vi "弹窗-创建设备选项.vi"() -> (3 "初始化的属性":T1[](array[typedef]))   [LabVIEW 2017]
panel:
  in  "发现的网络探头":string[](array[string])
  in  "标志-确定创建?":bool
  in  "发现的串口探头":u8[](array[numeric])
  in  "超时":i32
  out "扫描结果":string caption="新的设备"
  out "扫描进度":string
  in  "批量创建":u8=1 min=1 max=10
  in  "扫描探头":bool
  in  "探头类型":enum16{"网络探头", "串口探头"}(ring)
  in  "确定":bool
  in  "取消":bool
  out "信号-关闭窗口":bool=TRUE
  # "创建选项"
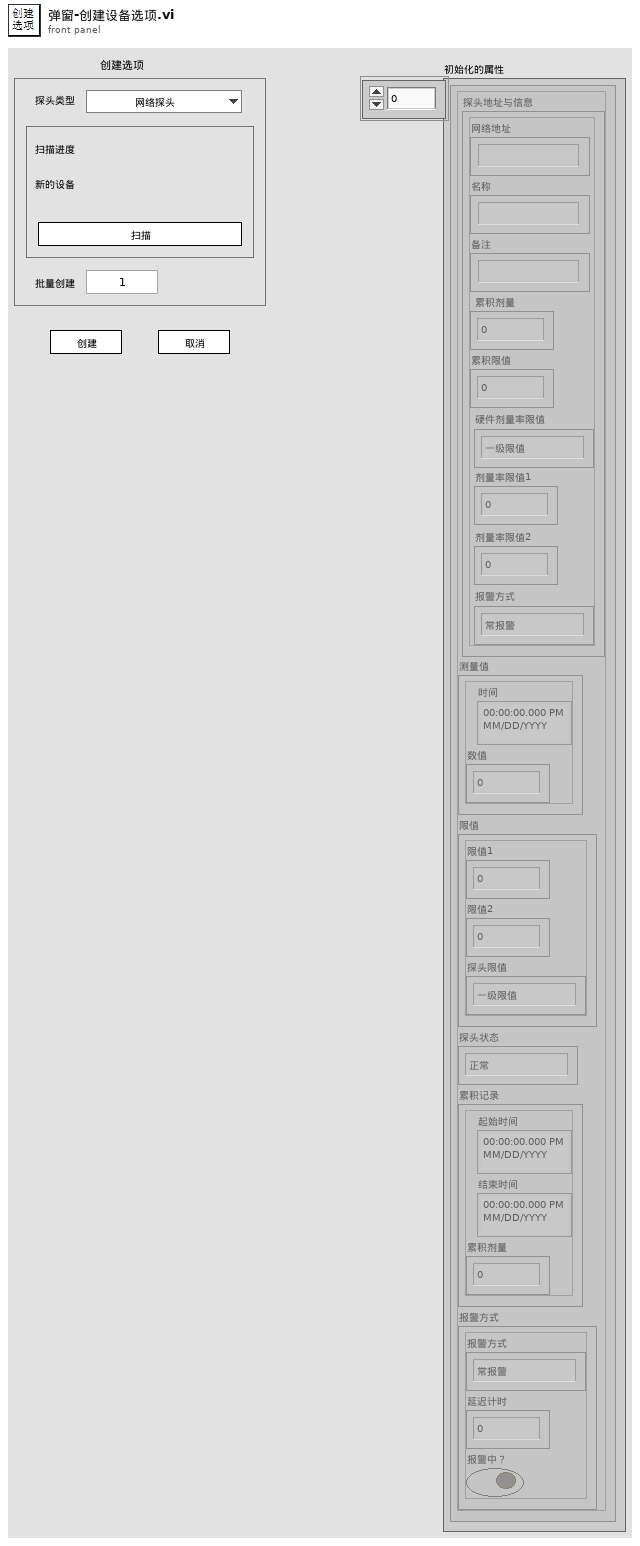
[diagram p1: front panel]
types:
  T1 = typedef "探头属性.ctl" = cluster{"探头地址与信息":T2, "测量值":T5, "限值":T6, "探头状态":T7, "累积记录":T8, "报警方式":T9}
  T2 = typedef "探测器信息.ctl" = cluster{"网络地址":string, "名称":string, "备注":string, "累积剂量":dbl, "累积限值":dbl, "硬件剂量率限值":T3, "剂量率限值1":dbl, "剂量率限值2":dbl, "报警方式":T4}
  T3 = typedef "探头剂量率限值选择.ctl" = enum16{"一级限值", "二级限值"}
  T4 = typedef "报警方式选择.ctl" = enum16{"常报警", "自动静音", "手动静音"}
  T5 = typedef "测量值.ctl" = cluster{"时间":timestamp, "数值":dbl}
  T6 = typedef "剂量率限值.ctl" = cluster{"限值1":dbl, "限值2":dbl, "探头限值":T3}
  T7 = typedef "探头状态.ctl" = enum16{"正常", "离线", "禁用", "一级报警", "二级报警", "累积报警"}
  T8 = typedef "单条累积记录.ctl" = cluster{"起始时间":timestamp, "结束时间":timestamp, "累积剂量":dbl}
  T9 = typedef "报警方式.ctl" = cluster{"报警方式":T4, "延迟计时":u16, "报警中？":bool}
  T10 = typedef "簇-输入.ctl" = cluster{"配置文件动作":T11, "数据输入":variant}
  T11 = typedef "枚举-配置文件动作.ctl" = enum16{"初始化加载配置", "读取配置", "写入-屏幕键盘", "写入-静音延迟", "写入-主要探头类型", "写入-串口配置", "写入-累积定时", "写入-导出定时", "保存配置到文件"}
  T12 = enum32{"Invalid", "Standard", "Closed", "Hidden", "Minimized", "Maximized"}
  T13 = enum8{"Enabled", "Disabled", "Disabled and Grayed Out"}
  T14 = typedef "枚举-主要探头类型.ctl" = enum16{"网络探头", "串口探头"}
  T15 = typedef "簇-配置文件内容.ctl" = cluster{"调试模式？":bool, "屏幕键盘？":bool, "软件版本":string, "静音延迟 s":u16, "主要探头类型":T14, "串口配置":cluster{"COM口":refnum<visa-resource-name>, "波特率":enum16{"9600", "19200"}, "读写超时ms":i16, "丢包判定次数":i16}, "定时配置-累积分段":T16, "定时配置-自动导出":cluster{"定时配置-自动导出":T16, "分别导出?":bool}}
  T16 = typedef "簇-定时配置.ctl" = cluster{"定时模式":enum16{"绝对时间", "相对时间"}, "单位":enum16{"年", "月", "日", "时", "分"}, "间隔":u8, "目标时刻":timestamp}
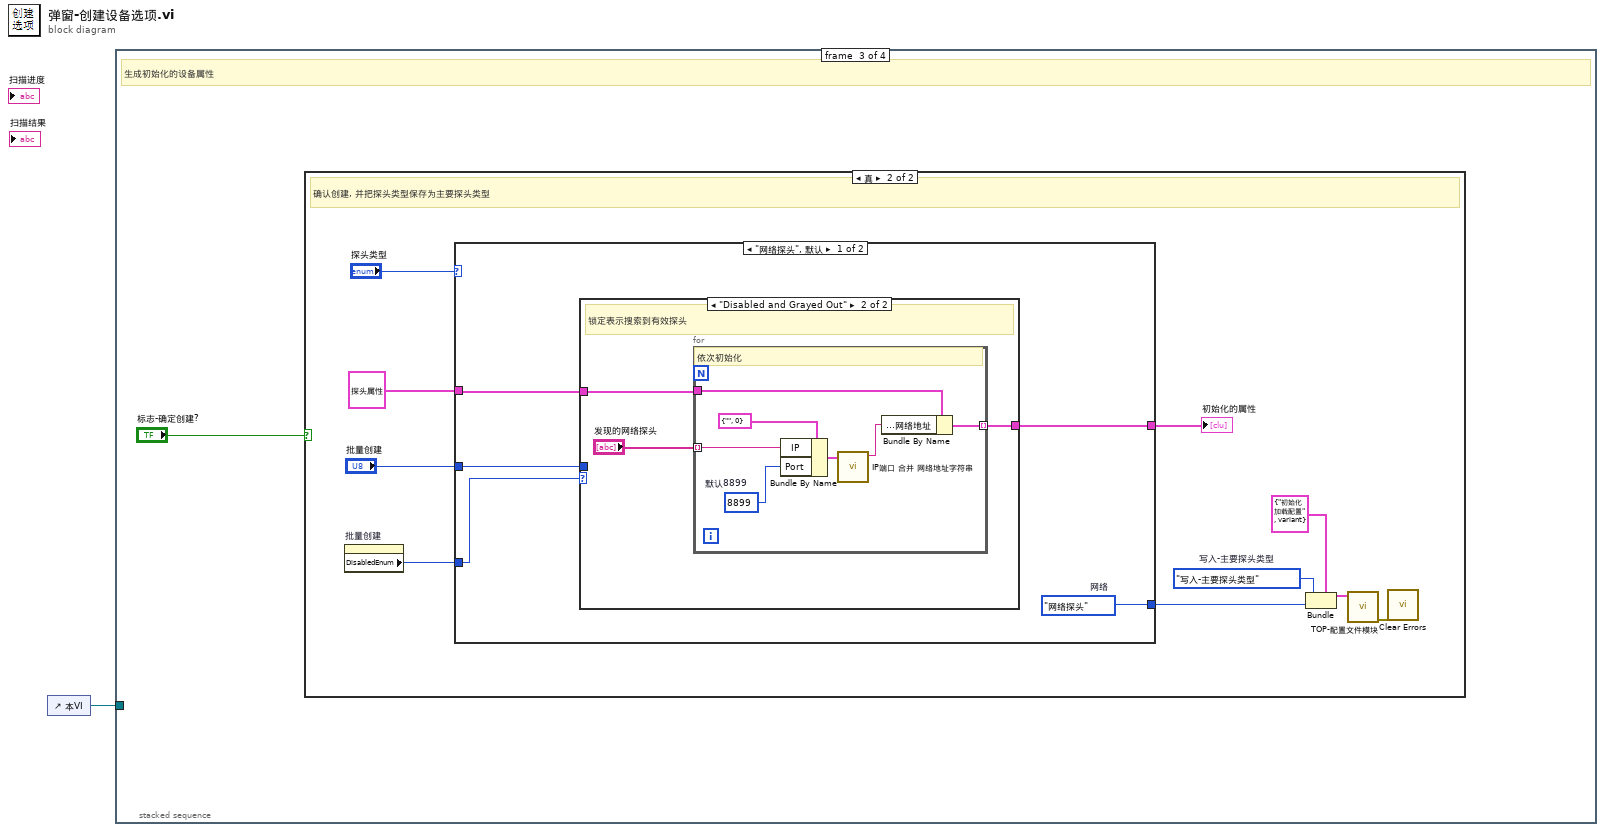
[diagram p0: block diagram]
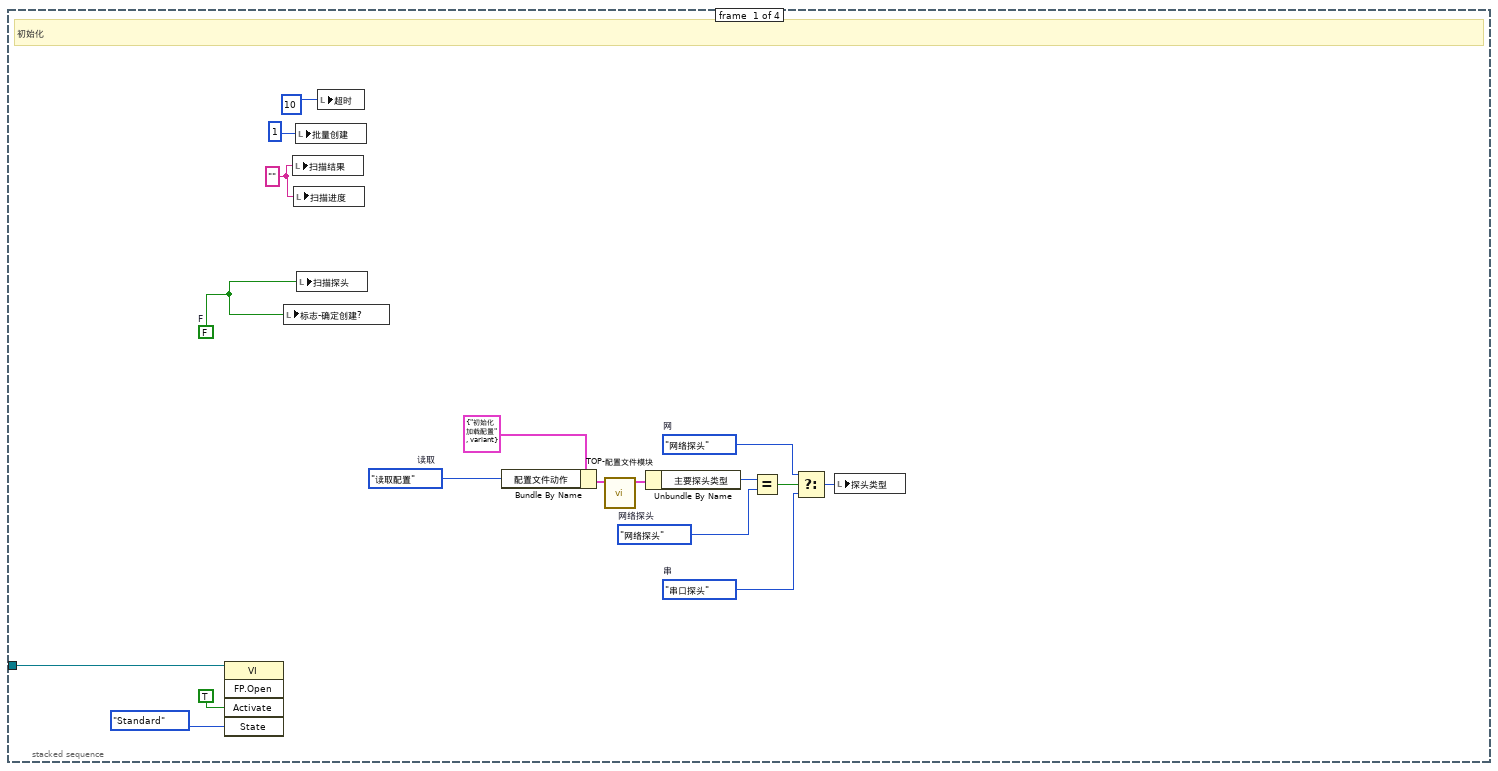
[diagram p2: hidden frame]
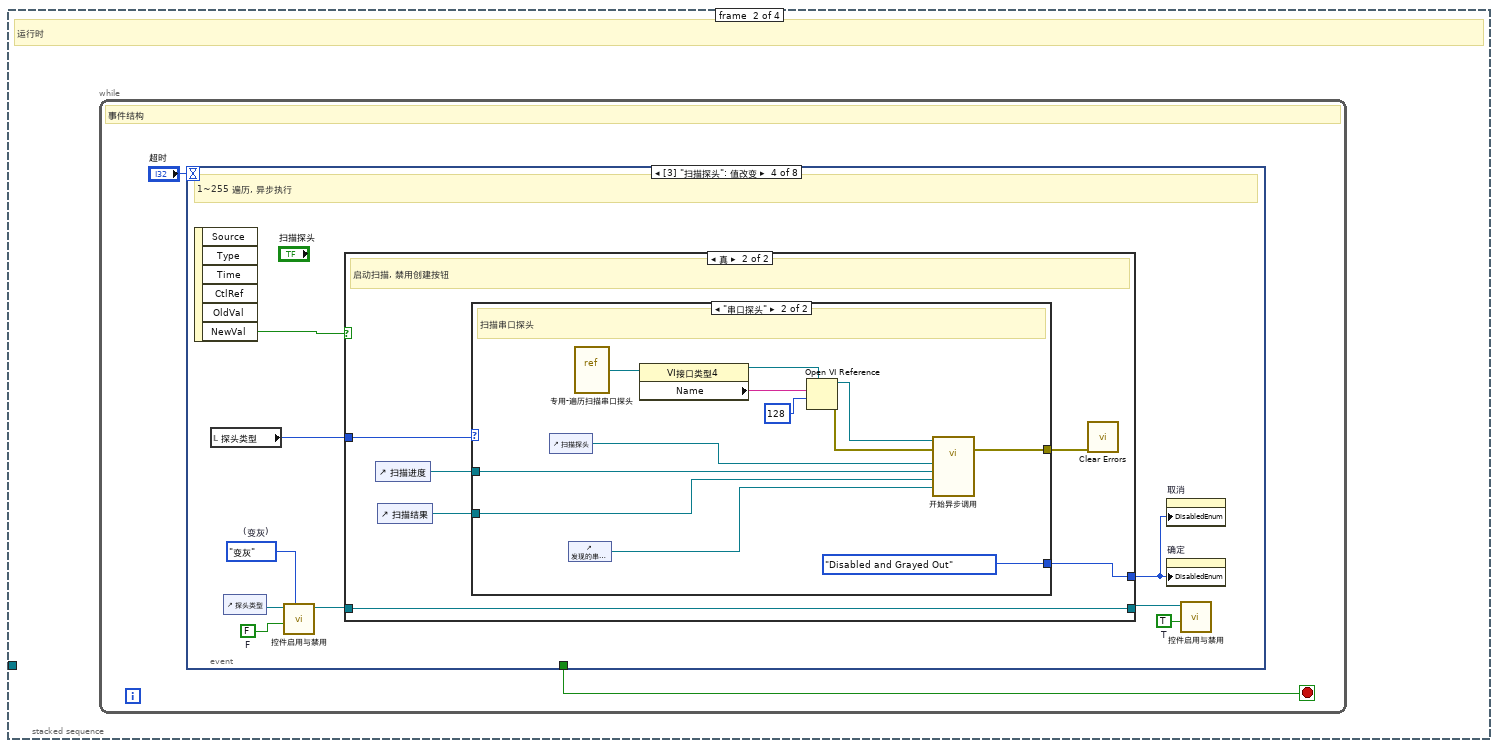
[diagram p3: hidden frame]
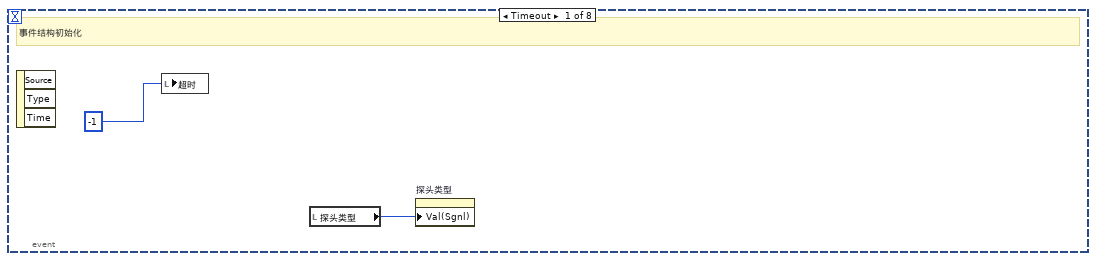
[diagram p4: hidden frame]
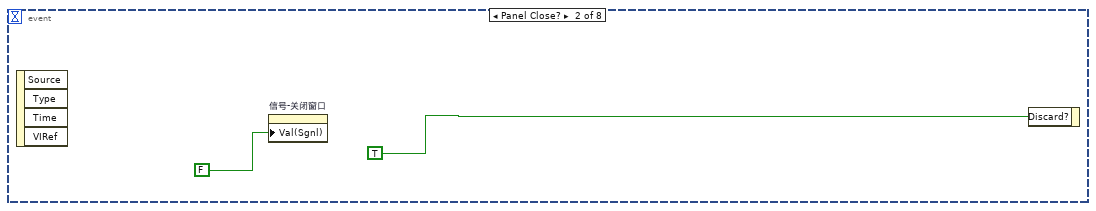
[diagram p5: hidden frame]
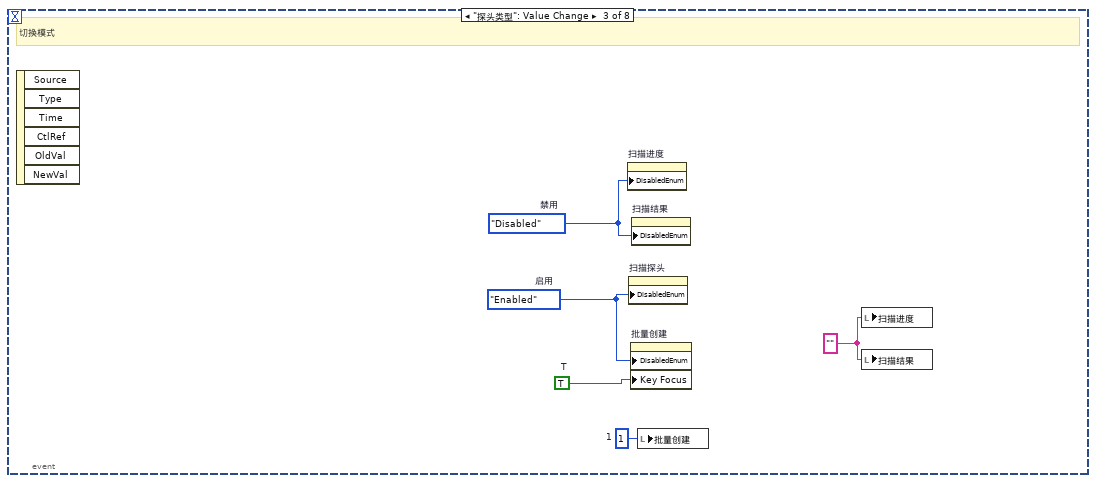
[diagram p6: hidden frame]
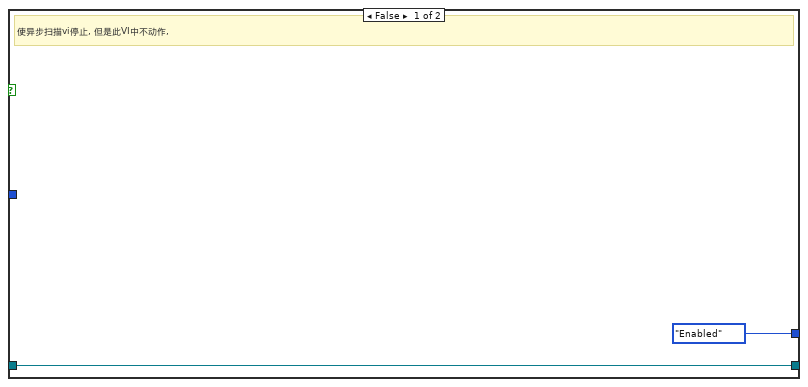
[diagram p7: hidden frame]
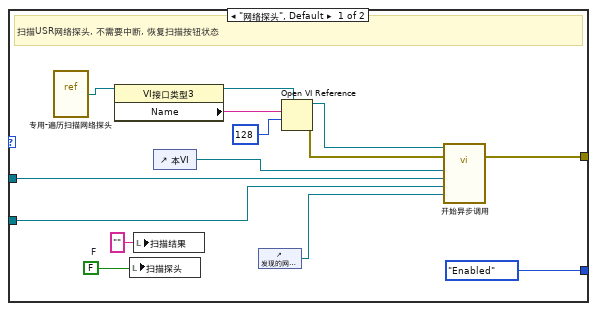
[diagram p8: hidden frame]
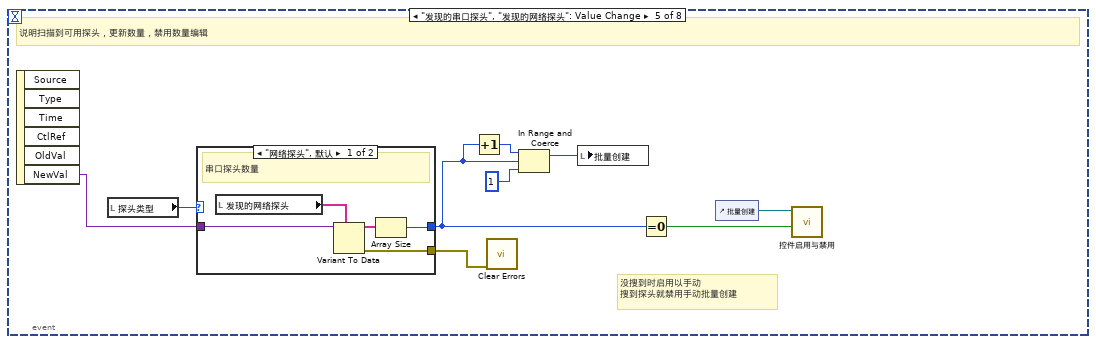
[diagram p9: hidden frame]
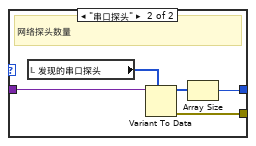
[diagram p10: hidden frame]
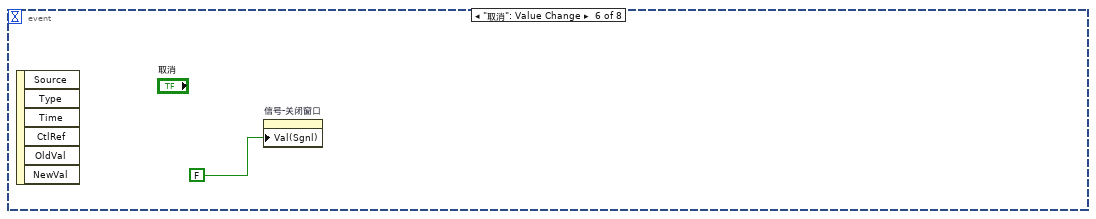
[diagram p11: hidden frame]
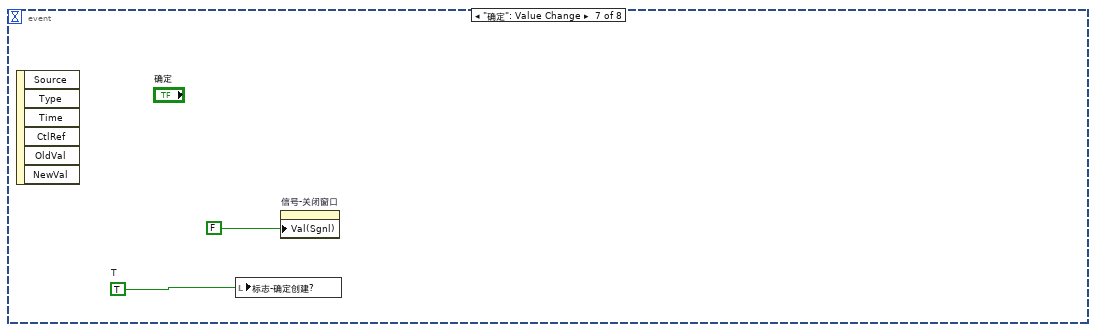
[diagram p12: hidden frame]
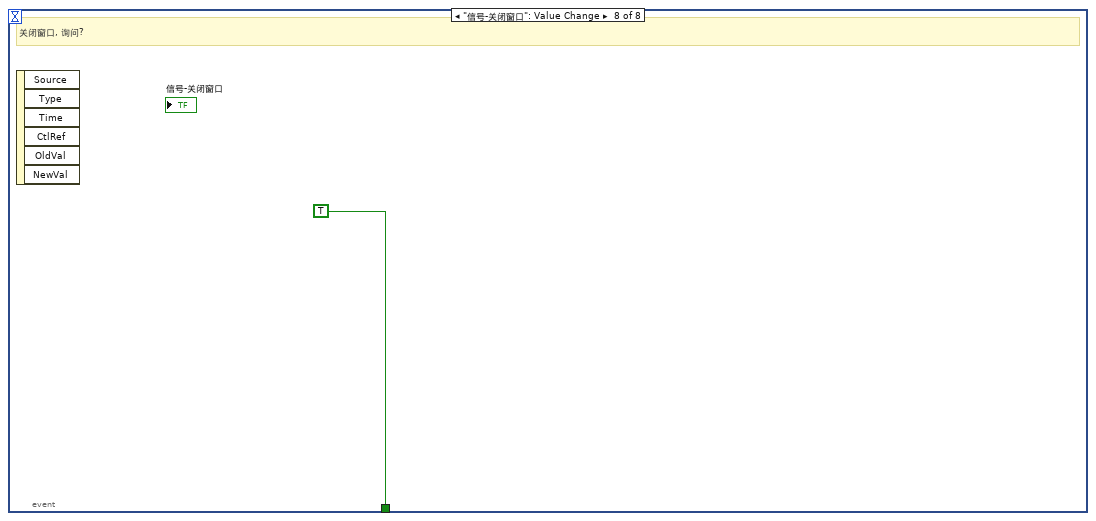
[diagram p13: hidden frame]
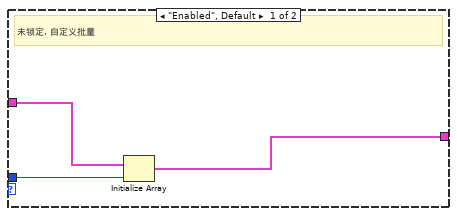
[diagram p15: hidden frame]
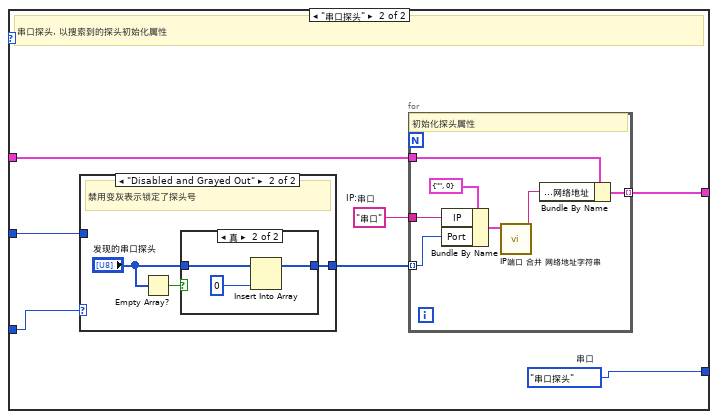
[diagram p16: hidden frame]
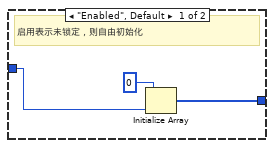
[diagram p17: hidden frame]
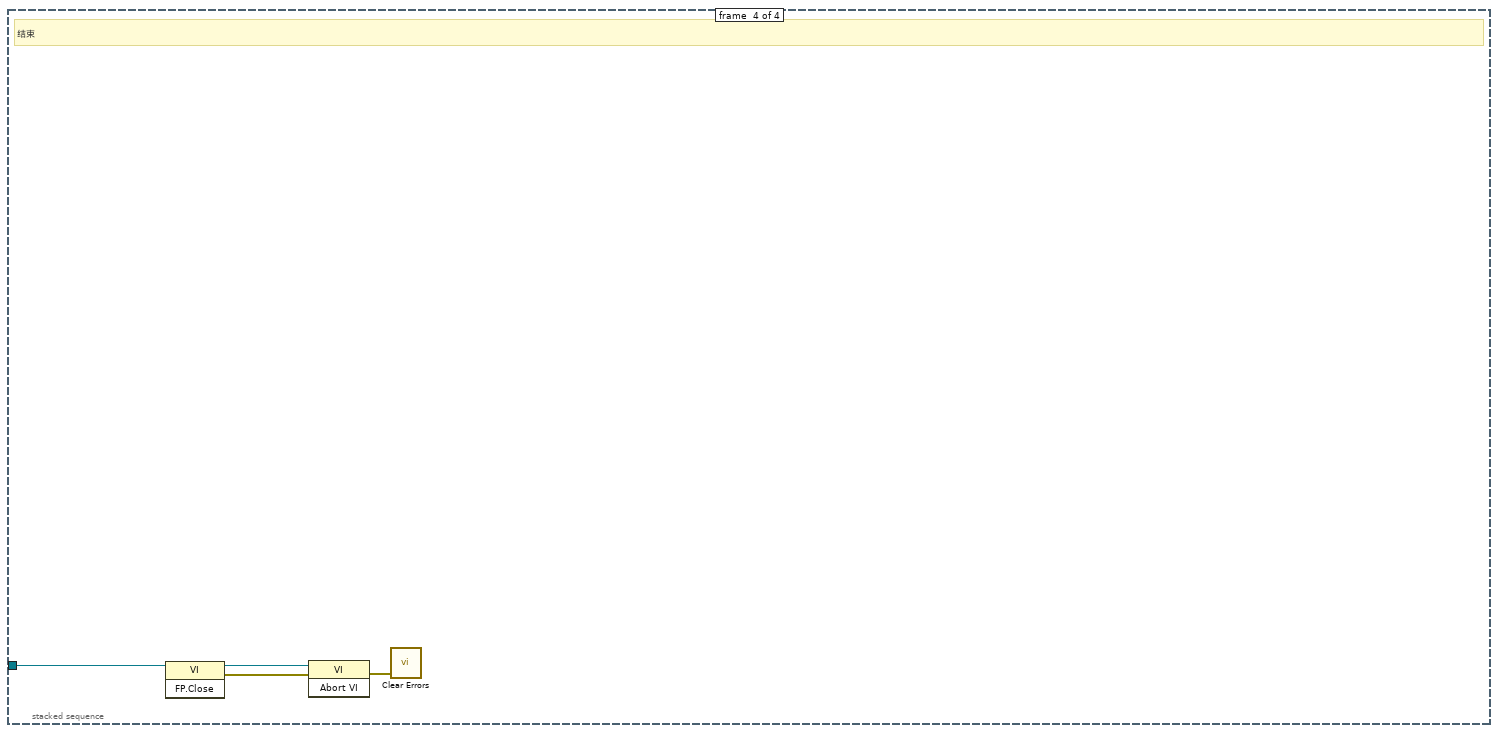
[diagram p19: hidden frame]
diagram:
  n1 = control-ref of="本VI"() -> (w1:refnum<vi>)
  n2 = stacked-sequence {
    tunnel: w1 -> [w18 _ _ w152]
    frame #0 {
      w2 = FALSE  # F
      w5 = enum16{"网络探头", "串口探头"}."串口探头"  # 串
      w6 = enum16{"网络探头", "串口探头"}."网络探头"  # 网
      w8 = 枚举-主要探头类型."网络探头"  # 网络探头
      w11 = 枚举-配置文件动作."读取配置"  # 读取
      w15 = "" ("扫描结果")
      # "初始化"
      n3 = invoke class="VI" method="FP.Open"(reference=w18, "Activate"=TRUE ("激活？"), "State"=T12."Standard" ("状态")) -> ()  [unwired: 2 in, 5 out]
      n4 = local write "标志-确定创建?"(w2) -> ()
      n5 = local write "扫描结果"(w15) -> ()
      n6 = local write "扫描进度"(w15) -> ()
      n7 = local write "批量创建"(u8 1 ("批量创建")) -> ()
      n8 = local write "扫描探头"(w2) -> ()
      n9 = local write "超时"(10 ("超时")) -> ()
      n10 = Bundle By Name(cluster=T10 {"配置文件动作"=enum."初始化加载配置", "数据输入"=variant} ("输入"), "配置文件动作"=w11) -> (w12:T10)
      n11 = call "TOP-配置文件模块.vi"("输入"=w12) -> ("配置文件"=w10:T15)  [unwired: 9 in, 1 out]
      n12 = Unbundle By Name(w10) -> ("主要探头类型"=w9:T14)
      n13 = Equal?(x=w9, y=w8) -> (x = y?=w7:bool)
      n14 = Select(t=w6, s=w7, f=w5) -> (s? t:f=w4:enum16{"网络探头", "串口探头"})
      n15 = local write "探头类型"(w4) -> ()
    }
    frame #1 {
      # "运行时"
      n16 = while {
        stop <- w20 stop-if-true
        # "事件结构"
        n17 = event shown="[3] \"扫描探头\": 值改变" {
          selector: _ -> [_ _ _ _ _ _ _ _]
          dyn-events: _ -> [_ _ _ _ _ _ _ _]
          timeout: "超时" -> [_ _ _ _ _ _ _ _]
          tunnel: [_ _ _ _ _ _ _ TRUE] -> w20
          event Timeout {
            # "事件结构初始化"
            n18 = event-data() -> ()  [unwired: 1 in, 3 out]
            n19 = local write "超时"(-1 ("超时")) -> ()
            n20 = local read "探头类型"() -> (w21:enum16{"网络探头", "串口探头"})
            n21 = property on="探头类型" class="Enum (严格)"("Val(Sgnl)"=w21) -> ()  [unwired: 2 in, 2 out]
          }
          event Panel Close? {
            n22 = event-data() -> ()  [unwired: 1 in, 4 out]
            n23 = property on="信号-关闭窗口" class="Bool (严格)"("Val(Sgnl)"=FALSE ("值(信号)")) -> ()  [unwired: 2 in, 2 out]
            n24 = event-data("Discard?"=TRUE ("放弃？")) -> ()  [unwired: 1 in, 1 out]
          }
          event "探头类型": Value Change {
            w25 = u8 1  # 1
            w29 = T13."Disabled"  # 禁用
            w26 = "" ("扫描进度")
            w27 = T13."Enabled"  # 启用
            w28 = TRUE  # T
            # "切换模式"
            n25 = event-data() -> ()  [unwired: 1 in, 6 out]
            n26 = property on="扫描进度" class="Str"("DisabledEnum"=w29) -> ()  [unwired: 2 in, 2 out]
            n27 = property on="扫描探头" class="Bool (严格)"("DisabledEnum"=w27) -> ()  [unwired: 2 in, 2 out]
            n28 = property on="批量创建" class="DigNum (严格)"("DisabledEnum"=w27, "Key Focus"=w28) -> ()  [unwired: 2 in, 2 out]
            n29 = property on="扫描结果" class="Str"("DisabledEnum"=w29) -> ()  [unwired: 2 in, 2 out]
            n30 = local write "批量创建"(w25) -> ()
            n31 = local write "扫描进度"(w26) -> ()
            n32 = local write "扫描结果"(w26) -> ()
          }
          event "扫描探头": Value Change {
            w30 = TRUE  # T
            w33 = enum16{"变灰", "不可见"}."变灰"  # (变灰)
            w34 = FALSE  # F
            # "1~255 遍历, 异步执行"
            n33 = event-data() -> ("NewVal"=w38:bool)  [unwired: 1 in, 5 out]
            n34 = local read "探头类型"() -> (w36:enum16{"网络探头", "串口探头"})
            n35 = control-ref of="探头类型"() -> (w35:refnum<vi>)
            n36 = call "控件启用与禁用.vi"("禁用效果(变灰)"=w33, "启用？"=w34, "控件引用"=w35) -> ("引用输出"=w32:refnum<vi>)  [unwired: 8 in]
            n37 = case shown="真" w38 {
              tunnel: [T13."Enabled" ("禁用") w44] -> w37
              tunnel: w36 -> [_ w46]
              tunnel: w32 -> [w39 w45]
              tunnel: [w39 w45] -> w31
              frame False {
                # "使异步扫描vi停止, 但是此VI中不动作,"
              }
              frame True {
                # "启动扫描, 禁用创建按钮"
                n38 = control-ref of="扫描进度"() -> (w43:refnum<vi>)
                n39 = control-ref of="扫描结果"() -> (w42:refnum<vi>)
                n40 = case shown="\"串口探头\"" w46 {
                  tunnel: [T13."Enabled" ("禁用") T13."Disabled and Grayed Out" ("禁用")] -> w44
                  tunnel: w43 -> [w50 w63]
                  tunnel: w42 -> [w49 w62]
                  tunnel: [w52 w61] -> w41
                  frame "网络探头", Default {
                    w59 = FALSE  # F
                    # "扫描USR网络探头, 不需要中断, 恢复扫描按钮状态"
                    n41 = vi-ref "专用-遍历扫描网络探头.vi"() -> (w55:refnum<vi>)
                    n42 = property class="VI接口类型3"(reference=w55) -> (reference out=w54:refnum<vi>, "Name"=w58:string)  [unwired: 1 in, 1 out]
                    n43 = local write "扫描探头"(w59) -> ()
                    n44 = local write "扫描结果"("" ("扫描结果")) -> ()
                    n45 = control-ref of="本VI"() -> (w51:refnum<vi>)
                    n46 = control-ref of="发现的网络探头"() -> (w48:refnum<vi>)
                    n47 = Open VI Reference(type specifier VI Refnum (for type only)=w54, vi path=w58, options=128 ("选项")) -> (vi reference=w57:refnum<vi>, error out=w53:errorcluster)  [unwired: 3 in]
                    n48 = call-by-ref "开始异步调用"(reference=w57, error in=w53, "发现的探头[]-引用"=w48, "扫描结果-引用"=w49, "扫描进度-引用"=w50, "忙碌VI"=w51) -> (error out=w52:errorcluster)  [unwired: 8 in, 1 out]
                  }
                  frame "串口探头" {
                    # "扫描串口探头"
                    n49 = control-ref of="扫描探头"() -> (w68:refnum<vi>)
                    n50 = control-ref of="发现的串口探头"() -> (w67:refnum<vi>)
                    n51 = vi-ref "专用-遍历扫描串口探头.vi"() -> (w72:refnum<vi>)
                    n52 = property class="VI接口类型4"(reference=w72) -> (reference out=w70:refnum<vi>, "Name"=w71:string)  [unwired: 1 in, 1 out]
                    n53 = Open VI Reference(type specifier VI Refnum (for type only)=w70, vi path=w71, options=128 ("选项")) -> (vi reference=w69:refnum<vi>, error out=w66:errorcluster)  [unwired: 3 in]
                    n54 = call-by-ref "开始异步调用"(reference=w69, error in=w66, "发现的探头[]-引用"=w67, "扫描结果-引用"=w62, "扫描进度-引用"=w63, "扫描按钮-引用"=w68) -> (error out=w61:errorcluster)  [unwired: 8 in, 1 out]
                  }
                }
                n55 = call <vilib>:"Clear Errors.vi"("error in (no error)"=w41) -> ()  [unwired: 5 in, 2 out]
              }
            }
            n56 = property on="取消" class="Bool"("DisabledEnum"=w37) -> ()  [unwired: 2 in, 2 out]
            n57 = property on="确定" class="Bool"("DisabledEnum"=w37) -> ()  [unwired: 2 in, 2 out]
            n58 = call "控件启用与禁用.vi"("启用？"=w30, "控件引用"=w31) -> ()  [unwired: 9 in, 1 out]
          }
          event "发现的串口探头", "发现的网络探头": Value Change {
            # "没搜到时启用以手动\n搜到探头就禁用手动批量创建"
            # "说明扫描到可用探头，更新数量，禁用数量编辑"
            n59 = event-data() -> ("NewVal"=w81:variant)  [unwired: 1 in, 5 out]
            n60 = local read "探头类型"() -> (w80:enum16{"网络探头", "串口探头"})
            n61 = case shown="\"网络探头\", 默认" w80 {
              tunnel: w81 -> [w86 w91]
              tunnel: [w83 w90] -> w74
              tunnel: [w82 w87] -> w79
              frame "网络探头", Default {
                # "串口探头数量"
                n62 = local read "发现的网络探头"() -> (w85:string[])
                n63 = Variant To Data(type=w85, Variant=w86) -> (data=w84:string[], error out=w82:errorcluster)  [unwired: 1 in]
                n64 = Array Size(array=w84) -> (size(s)=w83:i32)
              }
              frame "串口探头" {
                # "网络探头数量"
                n65 = local read "发现的串口探头"() -> (w89:u8[])
                n66 = Variant To Data(type=w89, Variant=w91) -> (data=w88:u8[], error out=w87:errorcluster)  [unwired: 1 in]
                n67 = Array Size(array=w88) -> (size(s)=w90:i32)
              }
            }
            n68 = Increment(x=w74) -> (x+1=w73:i32)
            n69 = call <vilib>:"Clear Errors.vi"("error in (no error)"=w79) -> ()  [unwired: 5 in, 2 out]
            n70 = In Range and Coerce(upper limit=w73, x=w74, lower limit=u8 1 ("下限")) -> (coerced(x)=w75:i32)  [unwired: 1 out]
            n71 = local write "批量创建"(w75) -> ()
            n72 = Equal To 0?(x=w74) -> (x = 0?=w77:bool)
            n73 = control-ref of="批量创建"() -> (w78:refnum<vi>)
            n74 = call "控件启用与禁用.vi"("启用？"=w77, "控件引用"=w78) -> ()  [unwired: 9 in, 1 out]
          }
          event "取消": Value Change {
            n75 = event-data() -> ()  [unwired: 1 in, 6 out]
            n76 = property on="信号-关闭窗口" class="Bool (严格)"("Val(Sgnl)"=FALSE ("值(信号)")) -> ()  [unwired: 2 in, 2 out]
          }
          event "确定": Value Change {
            w93 = TRUE  # T
            n77 = event-data() -> ()  [unwired: 1 in, 6 out]
            n78 = local write "标志-确定创建?"(w93) -> ()
            n79 = property on="信号-关闭窗口" class="Bool (严格)"("Val(Sgnl)"=FALSE ("值(信号)")) -> ()  [unwired: 2 in, 2 out]
          }
          event "信号-关闭窗口": Value Change {
            # "关闭窗口, 询问?"
            n80 = event-data() -> ()  [unwired: 1 in, 6 out]
          }
        }
      }
    }
    frame #2 {
      # "生成初始化的设备属性"
      n81 = case shown="真" "标志-确定创建?" {
        frame False {
        }
        frame True {
          w101 = 枚举-配置文件动作."写入-主要探头类型"  # 写入-主要探头类型
          # "确认创建, 并把探头类型保存为主要探头类型"
          n82 = property on="批量创建" class="DigNum (严格)"() -> ("DisabledEnum"=w98:T13)  [unwired: 2 in, 2 out]
          n83 = case shown="\"网络探头\", 默认" "探头类型" {
            tunnel: [w107 w130] -> w105
            tunnel: T1 {"探头地址与信息"={"网络地址"="", "名称"="", "备注"="", "累积剂量"=0.0, "累积限值"=0.0, "硬件剂量率限值"=enum."一级限值", "剂量率限值1"=0.0, "剂量率限值2"=0.0, "报警方式"=enum."常报警"}, "测量值"={"时间"=timestamp(0 s since 1904-01-01), "数值"=0.0}, "限值"={"限值1"=0.0, "限值2"=0.0, "探头限值"=enum."一级限值"}, "探头状态"=enum."正常", "累积记录"={"起始时间"=timestamp(0 s since 1904-01-01), "结束时间"=timestamp(0 s since 1904-01-01), "累积剂量"=0.0}, "报警方式"={"报警方式"=enum."常报警", "延迟计时"=0, "报警中？"=FALSE}} ("探头属性") -> [w108 w129]
            tunnel: "批量创建" -> [w109 w125]
            tunnel: [w111 w127] -> w99
            tunnel: w98 -> [w110 w126]
            frame "网络探头", Default {
              w111 = 枚举-主要探头类型."网络探头"  # 网络
              n84 = case shown="\"Disabled and Grayed Out\"" w110 {
                tunnel: w109 -> [w114 _]
                tunnel: w108 -> [w113 w116]
                tunnel: [w112 w115] -> w107
                frame "Enabled", Default {
                  # "未锁定, 自定义批量"
                  n85 = Initialize Array(w113, w114) -> (w112:T1[])
                }
                frame "Disabled and Grayed Out" {
                  # "锁定表示搜索到有效探头"
                  n86 = for {
                    tunnel: w116 -> [w124]
                    tunnel: "发现的网络探头" -> [w118] mode=indexing
                    tunnel: [w119] -> w115 mode=indexing
                    w121 = u16 8899  # 默认8899
                    # "依次初始化"
                    n87 = Bundle By Name(cluster=cluster{"IP":string, "Port":u16} {"IP"="", "Port"=0} ("IP端口"), "IP"=w118, "Port"=w121) -> (w123:cluster{"IP":string, "Port":u16})
                    n88 = call "IP端口 合并 网络地址字符串.vi"("IP端口"=w123) -> ("IP端口字符串"=w120:string)  [unwired: 10 in]
                    n89 = Bundle By Name(cluster=w124, "探头地址与信息.网络地址"=w120) -> (w119:T1)
                  }
                }
              }
            }
            frame "串口探头" {
              w127 = 枚举-主要探头类型."串口探头"  # 串口
              w131 = "串口"  # IP:串口
              # "串口探头, 以搜索到的探头初始化属性"
              n90 = case shown="\"Disabled and Grayed Out\"" w126 {
                tunnel: [w132 w136] -> w128
                tunnel: w125 -> [w133 _]
                frame "Enabled", Default {
                  # "启用表示未锁定，则自由初始化"
                  n91 = Initialize Array(u8 0 ("数值"), w133) -> (w132:u8[])
                }
                frame "Disabled and Grayed Out" {
                  # "禁用变灰表示锁定了探头号"
                  n92 = Empty Array?(array="发现的串口探头") -> (empty?=w137:bool)
                  n93 = case shown="真" w137 {
                    tunnel: [w138 w139] -> w136
                    tunnel: "发现的串口探头" -> [w138 w141]
                    frame False {
                    }
                    frame True {
                      n94 = Insert Into Array(array=w141, new element=u8 0 ("数值")) -> (w139:u8[])  [unwired: 1 in]
                    }
                  }
                }
              }
              n95 = for {
                tunnel: w128 -> [w146] mode=indexing
                tunnel: w131 -> [w145]
                tunnel: [w143] -> w130 mode=indexing
                tunnel: w129 -> [w142]
                # "初始化探头属性"
                n96 = Bundle By Name(cluster=cluster{"IP":string, "Port":u16} {"IP"="", "Port"=0} ("IP端口"), "IP"=w145, "Port"=w146) -> (w148:cluster{"IP":string, "Port":u16})
                n97 = call "IP端口 合并 网络地址字符串.vi"("IP端口"=w148) -> ("IP端口字符串"=w144:string)  [unwired: 10 in]
                n98 = Bundle By Name(cluster=w142, "探头地址与信息.网络地址"=w144) -> (w143:T1)
              }
            }
          }
          "初始化的属性" <- w105
          n99 = Bundle(cluster=T10 {"配置文件动作"=enum."初始化加载配置", "数据输入"=variant} ("输入"), "配置文件动作"=w101, "数据输入"=w99) -> (w102:T10)
          n100 = call "TOP-配置文件模块.vi"("输入"=w102) -> ("error out"=w97:errorcluster)  [unwired: 9 in, 1 out]
          n101 = call <vilib>:"Clear Errors.vi"("error in (no error)"=w97) -> ()  [unwired: 5 in, 2 out]
        }
      }
    }
    frame #3 {
      # "结束"
      n102 = invoke class="VI" method="FP.Close"(reference=w152) -> (reference out=w151:refnum<vi>, error out=w150:errorcluster)  [unwired: 2 in, 1 out]
      n103 = invoke class="VI" method="Abort VI"(reference=w151, error in=w150) -> (error out=w149:errorcluster)  [unwired: 1 in, 2 out]
      n104 = call <vilib>:"Clear Errors.vi"("error in (no error)"=w149) -> ()  [unwired: 5 in, 2 out]
    }
  }
